vi "Create_Tree_PN.vi"(4 "Triangles":T3[](array[typedef]), 5 "Sf":dbl=0.6, 6 "dq":dbl=0.3927, 7 "L0":dbl=1.0, 8 "Pad":dbl=1.01) -> (0 "Mesh bounds":T1, 1 "Node stack size history":i32[](array[numeric]), 2 "All nodes processed and processed without error":bool, 3 "TreeNodes out":T2[](array[typedef]))   [LabVIEW 2011]
uses:
  Triangle2D.ctl
  TreeNode2D.ctl
  TreeNode2D Input Cluster.ctl
  <vilib>/Utility/file.llb/Write To Spreadsheet File (I64).vi
panel:
  out "Node tree representation":cluster{dbl[], dbl[]}(graph)
  out "Node stack size history":i32[](graph)
  in  "stop":bool
  in  "TreeNodes":T2[](array[typedef])
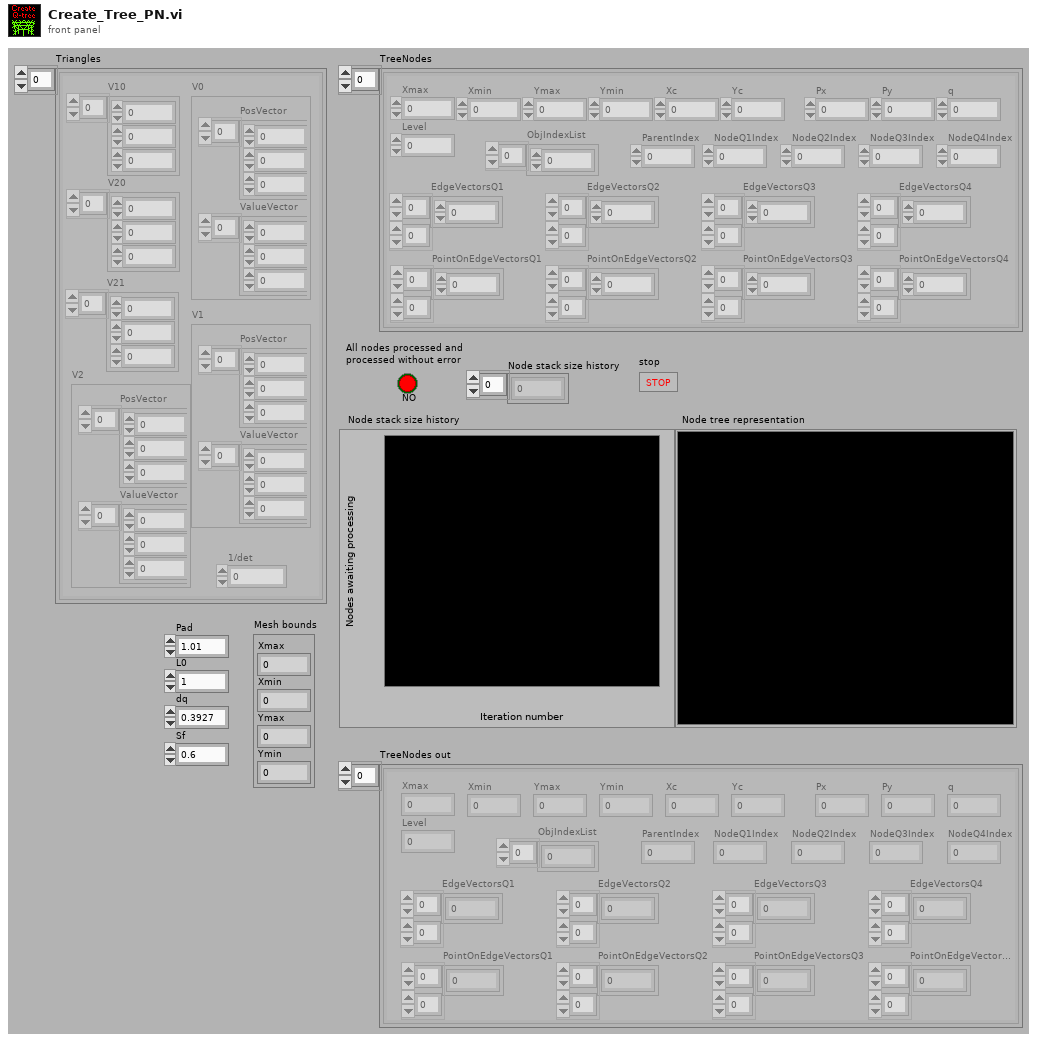
[diagram p1: front panel]
types:
  T1 = cluster{"Xmax":dbl, "Xmin":dbl, "Ymax":dbl, "Ymin":dbl}
  T2 = typedef "TreeNode2D.ctl" = cluster{"Xmax":dbl, "Xmin":dbl, "Ymax":dbl, "Ymin":dbl, "Xc":dbl, "Yc":dbl, "Px":dbl, "Py":dbl, "q":dbl, "Level":i32, "ObjIndexList":i32[], "ParentIndex":i32, "NodeQ1Index":i32, "NodeQ2Index":i32, "NodeQ3Index":i32, "NodeQ4Index":i32, "EdgeVectorsQ1":dbl[][], "EdgeVectorsQ2":dbl[][], "EdgeVectorsQ3":dbl[][], "EdgeVectorsQ4":dbl[][], "PointOnEdgeVectorsQ1":dbl[][], "PointOnEdgeVectorsQ2":dbl[][], "PointOnEdgeVectorsQ3":dbl[][], "PointOnEdgeVectorsQ4":dbl[][]}
  T3 = typedef "Triangle2D.ctl" = cluster{"V10":dbl[], "V20":dbl[], "1/det":dbl, "V0":cluster{"PosVector":dbl[], "ValueVector":dbl[]}, "V1":cluster{"PosVector":dbl[], "ValueVector":dbl[]}, "V2":cluster{"PosVector":dbl[], "ValueVector":dbl[]}, "V21":dbl[]}
  T4 = typedef "TreeNode2D Input Cluster.ctl" = cluster{"Xmax":dbl, "Xmin":dbl, "Ymax":dbl, "Ymin":dbl, "Xc":dbl, "Yc":dbl, "Px":dbl, "Py":dbl, "q":dbl, "Level":i32, "ObjIndexList":i32[], "ParentIndex":i32, "NodeQ1Index":i32, "NodeQ2Index":i32, "NodeQ3Index":i32, "NodeQ4Index":i32}
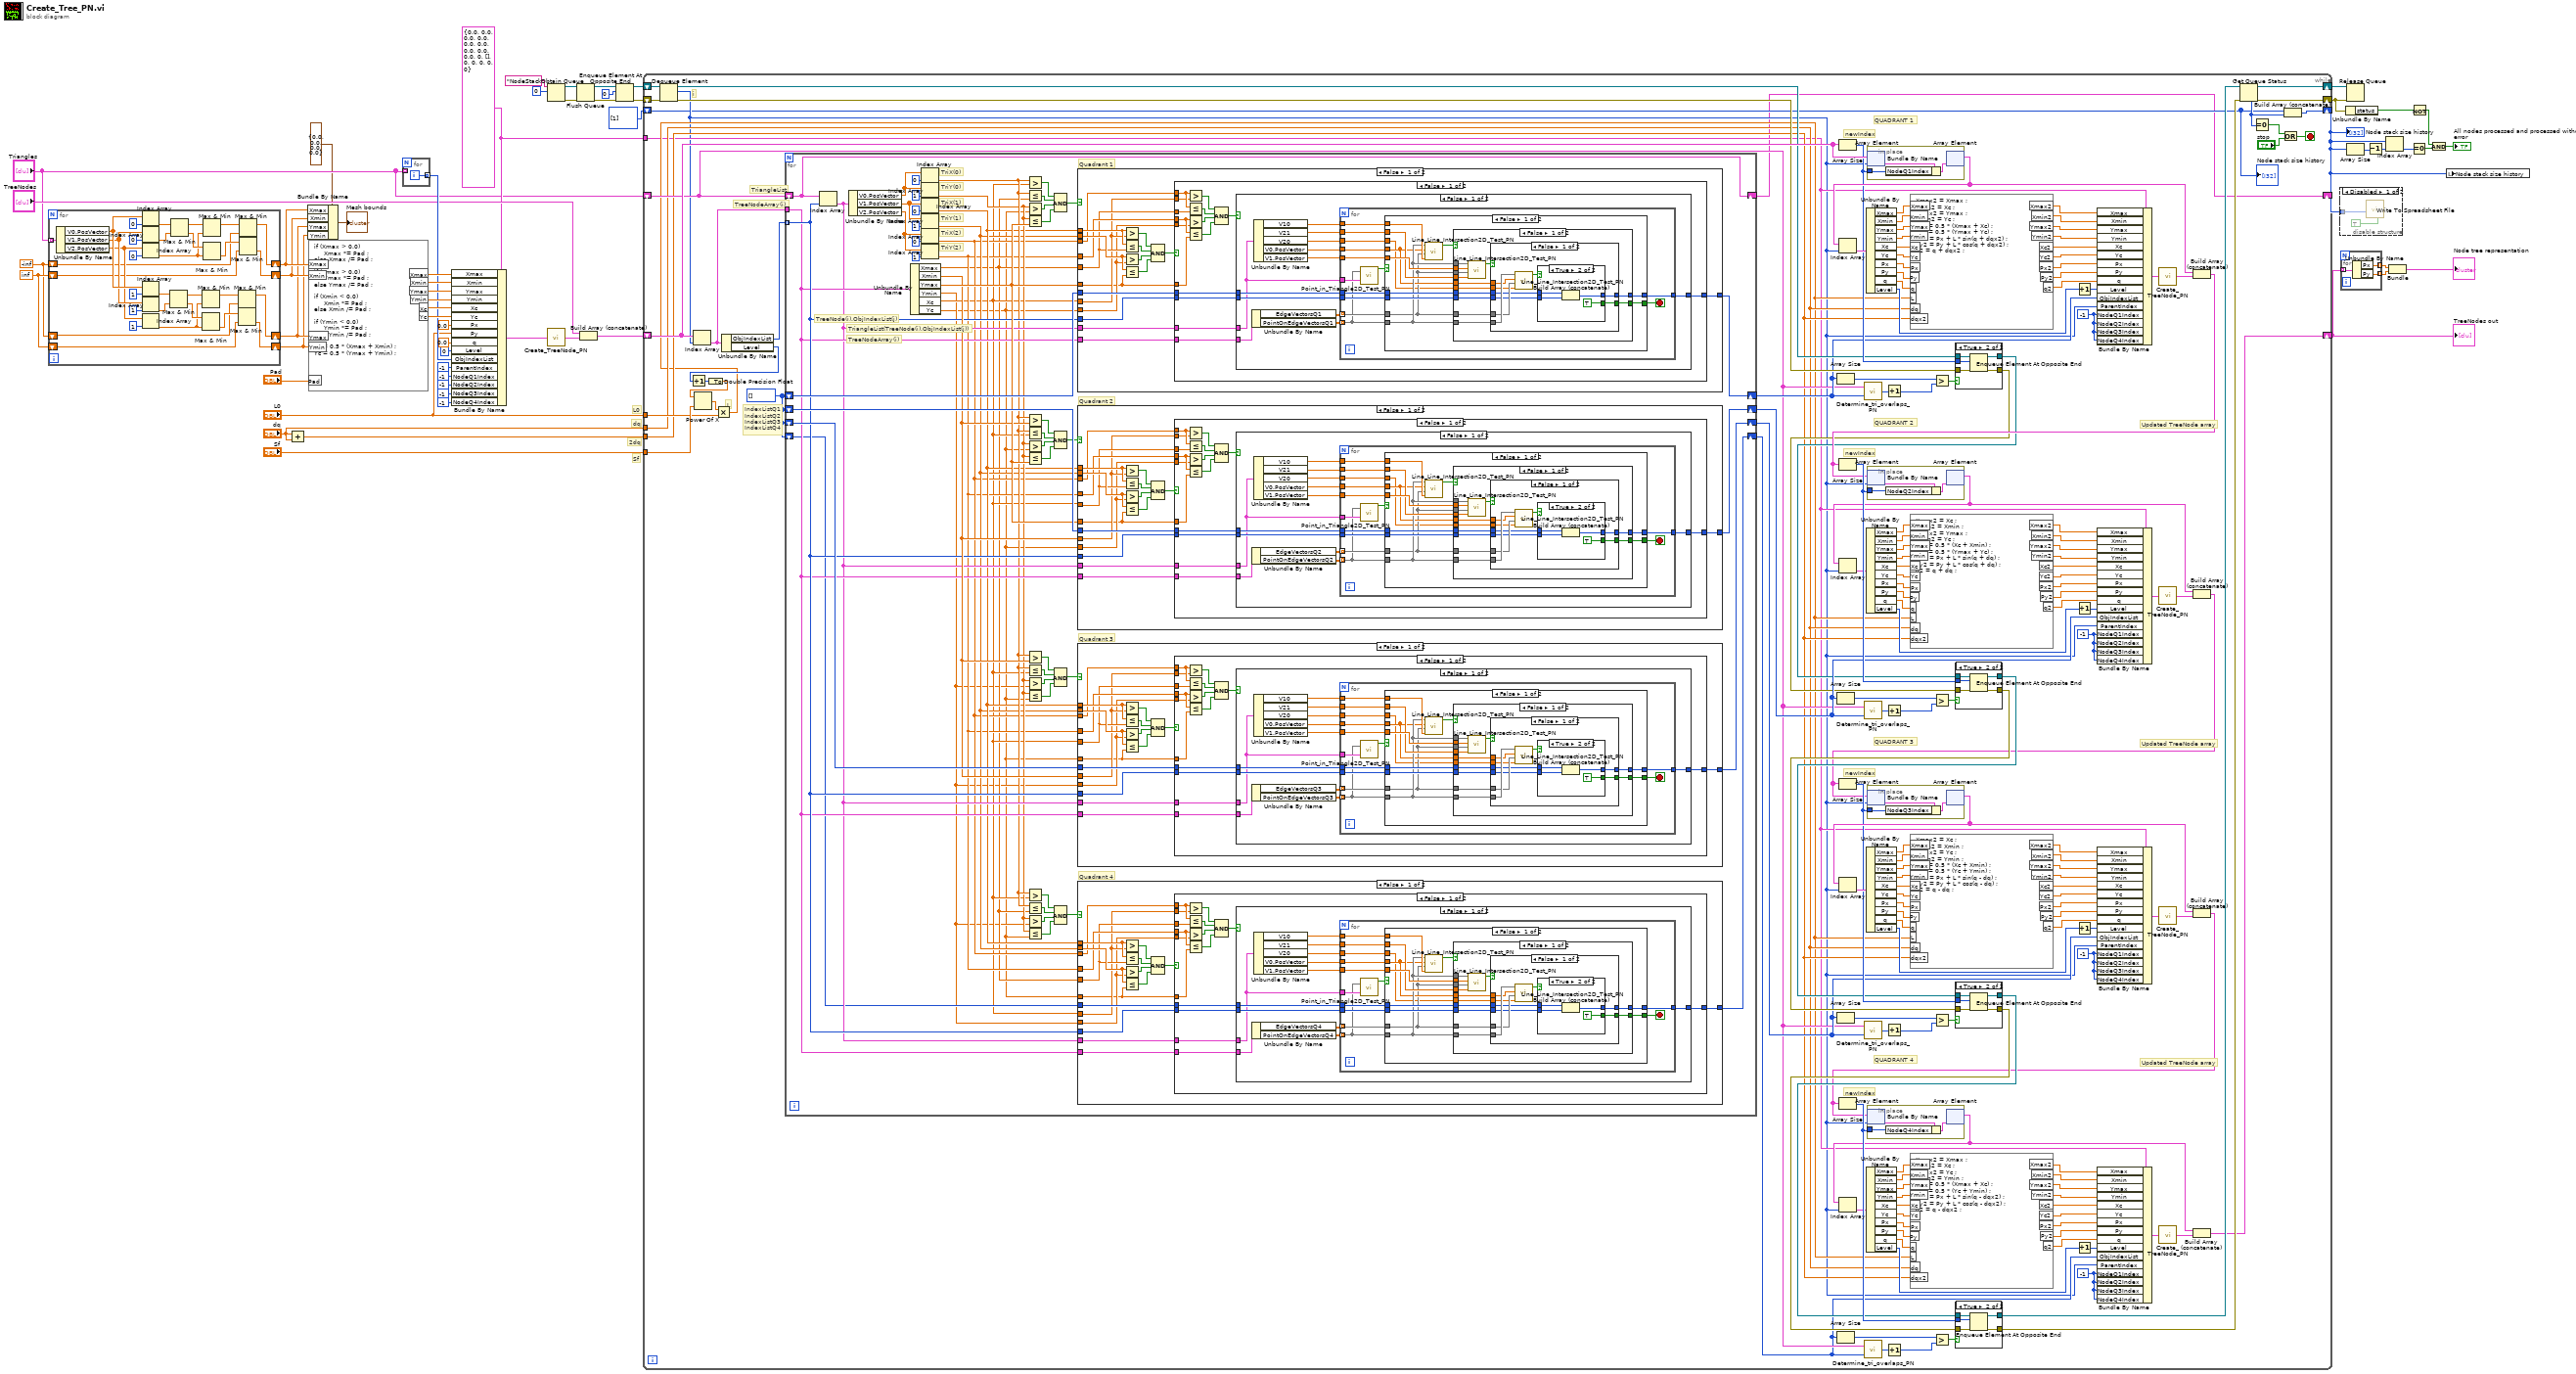
[diagram p0: block diagram]
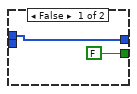
[diagram p7: hidden frame]
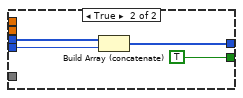
[diagram p8: hidden frame]
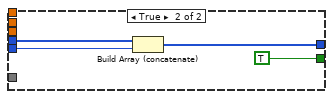
[diagram p9: hidden frame]
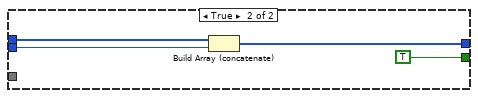
[diagram p10: hidden frame]
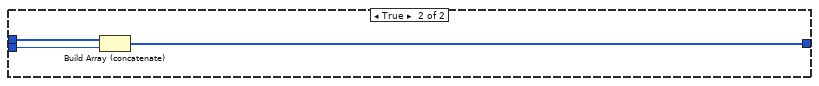
[diagram p11: hidden frame]
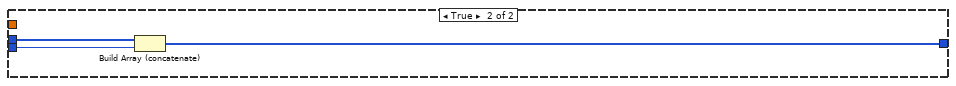
[diagram p12: hidden frame]
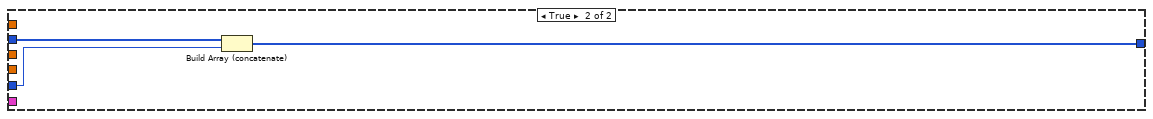
[diagram p13: hidden frame]
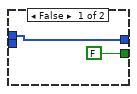
[diagram p14: hidden frame]
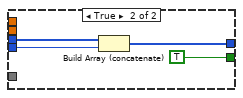
[diagram p15: hidden frame]
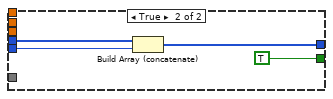
[diagram p16: hidden frame]
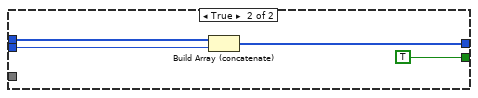
[diagram p17: hidden frame]
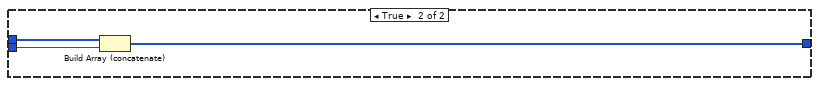
[diagram p18: hidden frame]
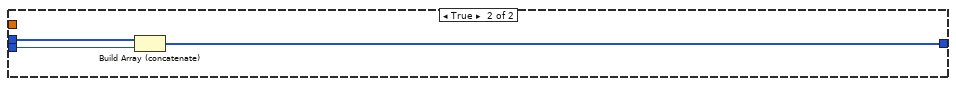
[diagram p19: hidden frame]
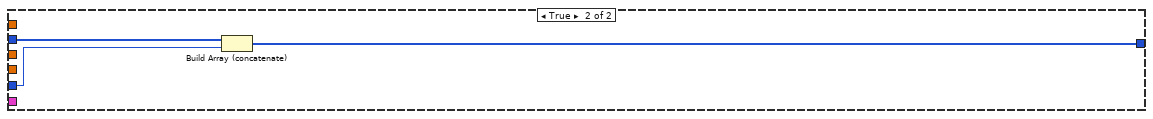
[diagram p20: hidden frame]
diagram:
  w8 = inf
  w7 = -inf
  w25 = T4 {"Xmax"=0.0, "Xmin"=0.0, "Ymax"=0.0, "Ymin"=0.0, "Xc"=0.0, "Yc"=0.0, "Px"=0.0, "Py"=0.0, "q"=0.0, "Level"=0, "ObjIndexList"=[], "ParentIndex"=0, "NodeQ1Index"=0, "NodeQ2Index"=0, "NodeQ3Index"=0, "NodeQ4Index"=0} ("Input cluster")
  # "Sf"
  # "L0"
  # "dq"
  # "2dq"
  n1 = for {
    tunnel: "Triangles" -> [w90] mode=indexing
    shift-right: [w72] -> w6
    shift-left: w7 -> [w73]
    shift-right: [w70] -> w5
    shift-left: w8 -> [w71]
    shift-right: [w60] -> w4
    shift-left: w7 -> [w62]
    shift-right: [w59] -> w3
    shift-left: w8 -> [w61]
    n2 = Unbundle By Name(w90) -> ("V0.PosVector"=w83:dbl[], "V1.PosVector"=w82:dbl[], "V2.PosVector"=w81:dbl[])
    n3 = Index Array(array=w83, index=0) -> (element=w80:dbl)
    n4 = Index Array(array=w82, index=0) -> (element=w79:dbl)
    n5 = Index Array(array=w81, index=0) -> (element=w76:dbl)
    n6 = Index Array(array=w83, index=1) -> (element=w65:dbl)
    n7 = Index Array(array=w82, index=1) -> (element=w64:dbl)
    n8 = Index Array(array=w81, index=1) -> (element=w63:dbl)
    n9 = Max & Min(x=w65, y=w64) -> (max(x,y)=w66:dbl, min(x,y)=w67:dbl)
    n10 = Max & Min(x=w80, y=w79) -> (max(x,y)=w78:dbl, min(x,y)=w77:dbl)
    n11 = Max & Min(x=w66, y=w63) -> (max(x,y)=w68:dbl)  [unwired: 1 out]
    n12 = Max & Min(x=w67, y=w63) -> (min(x,y)=w69:dbl)  [unwired: 1 out]
    n13 = Max & Min(x=w78, y=w76) -> (max(x,y)=w75:dbl)  [unwired: 1 out]
    n14 = Max & Min(x=w77, y=w76) -> (min(x,y)=w74:dbl)  [unwired: 1 out]
    n15 = Max & Min(x=w68, y=w62) -> (max(x,y)=w60:dbl)  [unwired: 1 out]
    n16 = Max & Min(x=w69, y=w61) -> (min(x,y)=w59:dbl)  [unwired: 1 out]
    n17 = Max & Min(x=w75, y=w73) -> (max(x,y)=w72:dbl)  [unwired: 1 out]
    n18 = Max & Min(x=w74, y=w71) -> (min(x,y)=w70:dbl)  [unwired: 1 out]
  }
  n19 = Add(x="dq", y="dq") -> (x+y=w27:dbl)
  n20 = Bundle By Name(cluster=T1 {"Xmax"=0.0, "Xmin"=0.0, "Ymax"=0.0, "Ymin"=0.0} ("Mesh bounds"), "Xmax"=w6, "Xmin"=w5, "Ymax"=w4, "Ymin"=w3) -> (→"Mesh bounds":T1)
  n21 = formula code="if (Xmax > 0.0)\n     Xmax *= Pad ;\nelse Xmax /= Pad ;\n\nif (Ymax > 0.0)\n     Ymax *= Pad ;\nelse Ymax /= Pad ;\n\nif (Xmin < 0.0)\n     Xmin *= Pad ;\nelse Xmin /= Pad ;\n\nif (Ymin < 0.0)\n     Ymin *= Pad ;\nelse Ymin /= Pad ;\n\nXc = 0.5 * (Xmax + Xmin) ;\nYc = 0.5 * (Ymax + Ymin) ;"("Xmax"=w6, "Xmin"=w5, "Ymax"=w4, "Ymin"=w3, "Pad"="Pad") -> ("Xmax"=w50:dbl, "Xmin"=w51:dbl, "Ymax"=w52:dbl, "Ymin"=w53:dbl, "Xc"=w55:dbl, "Yc"=w54:dbl)
  n22 = for {
    tunnel: "Triangles" -> [_] mode=indexing
    tunnel: [w91] -> w40 mode=indexing
    i -> [w91]
  }
  n23 = Bundle By Name(cluster=w25, "Xmax"=w50, "Xmin"=w51, "Ymax"=w52, "Ymin"=w53, "Xc"=w55, "Yc"=w54, "Px"=0.0, "Py"="L0", "q"=0.0, "Level"=0, "ObjIndexList"=w40, "ParentIndex"=-1, "NodeQ1Index"=-1, "NodeQ2Index"=-1, "NodeQ3Index"=-1, "NodeQ4Index"=-1) -> (w39:T4)
  n24 = Obtain Queue(name (unnamed)="NodeStack", element data type=0) -> (queue out=w37:refnum<queue>, error out=w38:errorcluster)  [unwired: 3 in, 1 out]
  n25 = call "Create_TreeNode_PN.vi"("Input cluster"=w39) -> ("TreeNode out"=w33:T2)
  n26 = Flush Queue(queue=w37, error in (no error)=w38) -> (queue out=w35:refnum<queue>, error out=w36:errorcluster)  [unwired: 1 out]
  n27 = Build Array (concatenate)("TreeNodes", w33) -> (w30:T2[])
  n28 = Enqueue Element At Opposite End(queue=w35, element=0, error in (no error)=w36) -> (queue out=w32:refnum<queue>, error out=w31:errorcluster)  [unwired: 2 out]
  n29 = while {
    shift-right: [w94] -> w11
    shift-left: w30 -> [w245]
    shift-right: [w253] -> w23
    shift-left: w31 -> [w256]
    shift-right: [w254] -> w29
    shift-left: w32 -> [w255]
    tunnel: "dq" -> [w107]
    tunnel: w27 -> [w108]
    tunnel: "L0" -> [w247]
    tunnel: "Sf" -> [w249]
    tunnel: w25 -> [w105]
    shift-right: [w99] -> w10
    shift-left: i32[] [1] -> [w93]
    shift-right: [w92] -> _
    shift-left: "Triangles" -> [w112]
    stop <- w97 stop-if-true
    w136 = -1 ("NodeQ1Index")
    w153 = -1 ("NodeQ1Index")
    w204 = -1 ("NodeQ1Index")
    w221 = -1 ("NodeQ1Index")
    w251 = i32[] []
    # "Updated TreeNode array"
    # "QUADRANT 4"
    # "newIndex"
    # "Updated TreeNode array"
    # "QUADRANT 3"
    # "newIndex"
    # "Updated TreeNode array"
    # "QUADRANT 2"
    # "newIndex"
    # "i"
    # "QUADRANT 1"
    # "newIndex"
    # "L"
    # "IndexListQ1\nIndexListQ2\nIndexListQ3\nIndexListQ4"
    # "TreeNodeArray(i)"
    # "TriangleList"
    n30 = Dequeue Element(queue=w255, error in (no error)=w256) -> (queue out=w216:refnum<queue>, element=w103:i32, error out=w215:errorcluster)  [unwired: 1 in, 1 out]
    n31 = Index Array(array=w245, index=w103) -> (element=w95:T2)
    n32 = Unbundle By Name(w95) -> ("ObjIndexList"=w252:i32[], "Level"=w250:i32)
    n33 = Increment(x=w250) -> (x+1=w246:i32)
    n34 = To Double Precision Float(number=w246) -> (double precision float=w213:dbl)
    n35 = Power Of X(1:w249, 2:w213) -> (0:w248:dbl)
    n36 = Multiply(x=w248, y=w247) -> (x*y=w106:dbl)
    n37 = for {
      tunnel: w95 -> [w316]
      tunnel: w252 -> [w317] mode=indexing
      shift-right: [w334] -> w211
      shift-left: w251 -> [w335]
      shift-right: [w332] -> w180
      shift-left: w251 -> [w333]
      shift-right: [w324] -> w143
      shift-left: w251 -> [w325]
      shift-right: [w298] -> w104
      shift-left: w251 -> [w314]
      shift-right: [w297] -> w92
      shift-left: w112 -> [w297]
      # "Quadrant 4"
      # "Quadrant 3"
      # "Quadrant 2"
      # "TreeNodeArray(i)"
      # "TriangleList(TreeNode(i).ObjIndexList(j))"
      # "TreeNode(i).ObjIndexList(j)"
      # "Quadrant 1"
      # "TriY(2)"
      # "TriX(2)"
      # "TriY(1)"
      # "TriX(1)"
      # "TriY(0)"
      # "TriX(0)"
      # "j"
      n38 = Index Array(array=w297, index=w317) -> (element=w315:T3)
      n39 = Unbundle By Name(w315) -> ("V0.PosVector"=w349:dbl[], "V1.PosVector"=w344:dbl[], "V2.PosVector"=w341:dbl[])
      n40 = Unbundle By Name(w316) -> ("Xmax"=w301:dbl, "Xmin"=w318:dbl, "Ymax"=w326:dbl, "Ymin"=w300:dbl, "Xc"=w302:dbl, "Yc"=w299:dbl)
      n41 = Index Array(array=w349, index=0) -> (element=w308:dbl)
      n42 = Index Array(array=w349, index=1) -> (element=w307:dbl)
      n43 = Index Array(array=w344, index=0) -> (element=w306:dbl)
      n44 = Index Array(array=w344, index=1) -> (element=w305:dbl)
      n45 = Index Array(array=w341, index=0) -> (element=w304:dbl)
      n46 = Index Array(array=w341, index=1) -> (element=w303:dbl)
      n47 = Greater?(x=w308, y=w302) -> (0:w340:bool)
      n48 = Less Or Equal?(x=w308, y=w301) -> (x <= y?=w339:bool)
      n49 = Greater?(x=w307, y=w299) -> (0:w338:bool)
      n50 = Less Or Equal?(x=w307, y=w326) -> (x <= y?=w337:bool)
      n51 = Greater?(x=w308, y=w318) -> (0:w328:bool)
      n52 = Less Or Equal?(x=w308, y=w302) -> (x <= y?=w329:bool)
      n53 = Greater?(x=w307, y=w299) -> (0:w330:bool)
      n54 = Less Or Equal?(x=w307, y=w326) -> (x <= y?=w331:bool)
      n55 = Greater?(x=w308, y=w318) -> (0:w323:bool)
      n56 = Less Or Equal?(x=w308, y=w302) -> (x <= y?=w322:bool)
      n57 = Greater?(x=w307, y=w300) -> (0:w321:bool)
      n58 = Less Or Equal?(x=w307, y=w299) -> (x <= y?=w320:bool)
      n59 = Greater?(x=w308, y=w302) -> (0:w310:bool)
      n60 = Less Or Equal?(x=w308, y=w301) -> (x <= y?=w311:bool)
      n61 = Greater?(x=w307, y=w300) -> (0:w312:bool)
      n62 = Less Or Equal?(x=w307, y=w299) -> (x <= y?=w313:bool)
      n63 = Compound Arithmetic op=AND(w340, w339, w338, w337) -> (w336:bool)
      n64 = Compound Arithmetic op=AND(w328, w329, w330, w331) -> (w327:bool)
      n65 = Compound Arithmetic op=AND(w323, w322, w321, w320) -> (w319:bool)
      n66 = Compound Arithmetic op=AND(w310, w311, w312, w313) -> (w309:bool)
      n67 = case shown="False" w336 {
        tunnel: w306 -> [w723 _]
        tunnel: w305 -> [w722 _]
        tunnel: w304 -> [w717 _]
        tunnel: w303 -> [w716 _]
        tunnel: w335 -> [w720 w829]
        tunnel: [w718 w828] -> w334
        tunnel: w317 -> [w719 w827]
        tunnel: w302 -> [w714 _]
        tunnel: w299 -> [w713 _]
        tunnel: w326 -> [w712 _]
        tunnel: w301 -> [w715 _]
        tunnel: w315 -> [w710 _]
        tunnel: w316 -> [w711 _]
        frame False {
          n68 = Greater?(x=w723, y=w714) -> (0:w724:bool)
          n69 = Less Or Equal?(x=w723, y=w715) -> (x <= y?=w725:bool)
          n70 = Greater?(x=w722, y=w713) -> (0:w726:bool)
          n71 = Less Or Equal?(x=w722, y=w712) -> (x <= y?=w727:bool)
          n72 = Compound Arithmetic op=AND(w724, w725, w726, w727) -> (w721:bool)
          n73 = case shown="False" w721 {
            tunnel: w720 -> [w731 w826]
            tunnel: w719 -> [w730 w825]
            tunnel: [w732 w824] -> w718
            tunnel: w717 -> [w739 _]
            tunnel: w716 -> [w738 _]
            tunnel: w715 -> [w737 _]
            tunnel: w714 -> [w736 _]
            tunnel: w713 -> [w735 _]
            tunnel: w712 -> [w734 _]
            tunnel: w711 -> [w729 _]
            tunnel: w710 -> [w728 _]
            frame False {
              n74 = Greater?(x=w739, y=w736) -> (0:w743:bool)
              n75 = Less Or Equal?(x=w739, y=w737) -> (x <= y?=w742:bool)
              n76 = Greater?(x=w738, y=w735) -> (0:w741:bool)
              n77 = Less Or Equal?(x=w738, y=w734) -> (x <= y?=w740:bool)
              n78 = Compound Arithmetic op=AND(w743, w742, w741, w740) -> (w733:bool)
              n79 = case shown="False" w733 {
                tunnel: [w745 w823] -> w732
                tunnel: w731 -> [w747 w822]
                tunnel: w730 -> [w746 w821]
                tunnel: w729 -> [w755 _]
                tunnel: w728 -> [w744 _]
                frame False {
                  n80 = Unbundle By Name(w755) -> ("EdgeVectorsQ1"=w754:dbl[][], "PointOnEdgeVectorsQ1"=w748:dbl[][])
                  n81 = Unbundle By Name(w744) -> ("V10"=w753:dbl[], "V21"=w752:dbl[], "V20"=w751:dbl[], "V0.PosVector"=w750:dbl[], "V1.PosVector"=w749:dbl[])
                  n82 = for {
                    tunnel: w754 -> [w762] mode=indexing
                    tunnel: w753 -> [w756]
                    tunnel: w752 -> [w757]
                    tunnel: w751 -> [w758]
                    tunnel: w750 -> [w759]
                    tunnel: w749 -> [w760]
                    tunnel: w748 -> [w761] mode=indexing
                    tunnel: w747 -> [w768]
                    tunnel: w746 -> [w767]
                    tunnel: [w766] -> w745
                    tunnel: w744 -> [w764]
                    stop <- w765 stop-if-true
                    n83 = call "Point_in_Triangle2D_Test_PN.vi"("2D Point to Test"=w761, "Triangle2D"=w764) -> ("Point is in triangle"=w763:bool)  [unwired: 3 out]
                    n84 = case shown="False" w763 {
                      tunnel: w768 -> [w776 w820]
                      tunnel: w767 -> [w775 w819]
                      tunnel: [w777 w818] -> w766
                      tunnel: [w778 TRUE] -> w765
                      tunnel: w762 -> [w770 _]
                      tunnel: w761 -> [w772 _]
                      tunnel: w760 -> [w774 _]
                      tunnel: w759 -> [w771 _]
                      tunnel: w758 -> [w769 _]
                      tunnel: w757 -> [w773 _]
                      tunnel: w756 -> [w780 _]
                      frame False {
                        n85 = call "Line_Line_Intersection2D_Test_PN.vi"("2D Dir. Vect. of Line 2 (not unit)"=w780, "2D Dir. Vect. of Line 1 (not unit)"=w770, "2D Point on Line 2"=w771, "2D Point on Line 1"=w772) -> ("Lines Intersect"=w779:bool)  [unwired: 2 out]
                        n86 = case shown="False" w779 {
                          tunnel: [w788 TRUE] -> w778
                          tunnel: [w785 w815] -> w777
                          tunnel: w776 -> [w787 w814]
                          tunnel: w775 -> [w786 w813]
                          tunnel: w772 -> [w793 _]
                          tunnel: w774 -> [w792 _]
                          tunnel: w770 -> [w791 _]
                          tunnel: w773 -> [w790 _]
                          tunnel: w772 -> [w784 _]
                          tunnel: w771 -> [w783 _]
                          tunnel: w770 -> [w782 _]
                          tunnel: w769 -> [w781 _]
                          frame False {
                            n87 = call "Line_Line_Intersection2D_Test_PN.vi"("2D Dir. Vect. of Line 2 (not unit)"=w790, "2D Dir. Vect. of Line 1 (not unit)"=w791, "2D Point on Line 2"=w792, "2D Point on Line 1"=w793) -> ("Lines Intersect"=w789:bool)  [unwired: 2 out]
                            n88 = case shown="False" w789 {
                              tunnel: [w797 TRUE] -> w788
                              tunnel: w787 -> [w796 w811]
                              tunnel: w786 -> [w795 w810]
                              tunnel: [w794 w809] -> w785
                              tunnel: w784 -> [w802 _]
                              tunnel: w783 -> [w801 _]
                              tunnel: w782 -> [w800 _]
                              tunnel: w781 -> [w799 _]
                              frame False {
                                n89 = call "Line_Line_Intersection2D_Test_PN.vi"("2D Dir. Vect. of Line 2 (not unit)"=w799, "2D Dir. Vect. of Line 1 (not unit)"=w800, "2D Point on Line 2"=w801, "2D Point on Line 1"=w802) -> ("Lines Intersect"=w798:bool)  [unwired: 2 out]
                                n90 = case shown="True" w798 {
                                tunnel: [FALSE TRUE] -> w797
                                tunnel: w796 -> [w804 w807]
                                tunnel: w795 -> [_ w806]
                                tunnel: [w804 w805] -> w794
                                frame False {
                                }
                                frame True {
                                n91 = Build Array (concatenate)(w807, w806) -> (w805:i32[])
                                }
                                }
                              }
                              frame True {
                                n92 = Build Array (concatenate)(w811, w810) -> (w809:i32[])
                              }
                            }
                          }
                          frame True {
                            n93 = Build Array (concatenate)(w814, w813) -> (w815:i32[])
                          }
                        }
                      }
                      frame True {
                        n94 = Build Array (concatenate)(w820, w819) -> (w818:i32[])
                      }
                    }
                  }
                }
                frame True {
                  n95 = Build Array (concatenate)(w822, w821) -> (w823:i32[])
                }
              }
            }
            frame True {
              n96 = Build Array (concatenate)(w826, w825) -> (w824:i32[])
            }
          }
        }
        frame True {
          n97 = Build Array (concatenate)(w829, w827) -> (w828:i32[])
        }
      }
      n98 = case shown="False" w327 {
        tunnel: w306 -> [w603 _]
        tunnel: w305 -> [w602 _]
        tunnel: w304 -> [w597 _]
        tunnel: w303 -> [w596 _]
        tunnel: w333 -> [w600 w709]
        tunnel: [w598 w708] -> w332
        tunnel: w317 -> [w599 w707]
        tunnel: w318 -> [w594 _]
        tunnel: w299 -> [w593 _]
        tunnel: w326 -> [w592 _]
        tunnel: w302 -> [w595 _]
        tunnel: w315 -> [w590 _]
        tunnel: w316 -> [w591 _]
        frame False {
          n99 = Greater?(x=w603, y=w594) -> (0:w604:bool)
          n100 = Less Or Equal?(x=w603, y=w595) -> (x <= y?=w605:bool)
          n101 = Greater?(x=w602, y=w593) -> (0:w606:bool)
          n102 = Less Or Equal?(x=w602, y=w592) -> (x <= y?=w607:bool)
          n103 = Compound Arithmetic op=AND(w604, w605, w606, w607) -> (w601:bool)
          n104 = case shown="False" w601 {
            tunnel: w600 -> [w611 w706]
            tunnel: w599 -> [w610 w705]
            tunnel: [w612 w704] -> w598
            tunnel: w597 -> [w619 _]
            tunnel: w596 -> [w618 _]
            tunnel: w595 -> [w617 _]
            tunnel: w594 -> [w616 _]
            tunnel: w593 -> [w615 _]
            tunnel: w592 -> [w614 _]
            tunnel: w591 -> [w609 _]
            tunnel: w590 -> [w608 _]
            frame False {
              n105 = Greater?(x=w619, y=w616) -> (0:w623:bool)
              n106 = Less Or Equal?(x=w619, y=w617) -> (x <= y?=w622:bool)
              n107 = Greater?(x=w618, y=w615) -> (0:w621:bool)
              n108 = Less Or Equal?(x=w618, y=w614) -> (x <= y?=w620:bool)
              n109 = Compound Arithmetic op=AND(w623, w622, w621, w620) -> (w613:bool)
              n110 = case shown="False" w613 {
                tunnel: [w625 w703] -> w612
                tunnel: w611 -> [w627 w702]
                tunnel: w610 -> [w626 w701]
                tunnel: w609 -> [w635 _]
                tunnel: w608 -> [w624 _]
                frame False {
                  n111 = Unbundle By Name(w635) -> ("EdgeVectorsQ2"=w634:dbl[][], "PointOnEdgeVectorsQ2"=w628:dbl[][])
                  n112 = Unbundle By Name(w624) -> ("V10"=w633:dbl[], "V21"=w632:dbl[], "V20"=w631:dbl[], "V0.PosVector"=w630:dbl[], "V1.PosVector"=w629:dbl[])
                  n113 = for {
                    tunnel: w634 -> [w642] mode=indexing
                    tunnel: w633 -> [w636]
                    tunnel: w632 -> [w637]
                    tunnel: w631 -> [w638]
                    tunnel: w630 -> [w639]
                    tunnel: w629 -> [w640]
                    tunnel: w628 -> [w641] mode=indexing
                    tunnel: w627 -> [w648]
                    tunnel: w626 -> [w647]
                    tunnel: [w646] -> w625
                    tunnel: w624 -> [w644]
                    stop <- w645 stop-if-true
                    n114 = call "Point_in_Triangle2D_Test_PN.vi"("2D Point to Test"=w641, "Triangle2D"=w644) -> ("Point is in triangle"=w643:bool)  [unwired: 3 out]
                    n115 = case shown="False" w643 {
                      tunnel: w648 -> [w656 w700]
                      tunnel: w647 -> [w655 w699]
                      tunnel: [w657 w698] -> w646
                      tunnel: [w658 TRUE] -> w645
                      tunnel: w642 -> [w650 _]
                      tunnel: w641 -> [w652 _]
                      tunnel: w640 -> [w654 _]
                      tunnel: w639 -> [w651 _]
                      tunnel: w638 -> [w649 _]
                      tunnel: w637 -> [w653 _]
                      tunnel: w636 -> [w660 _]
                      frame False {
                        n116 = call "Line_Line_Intersection2D_Test_PN.vi"("2D Dir. Vect. of Line 2 (not unit)"=w660, "2D Dir. Vect. of Line 1 (not unit)"=w650, "2D Point on Line 2"=w651, "2D Point on Line 1"=w652) -> ("Lines Intersect"=w659:bool)  [unwired: 2 out]
                        n117 = case shown="False" w659 {
                          tunnel: [w668 TRUE] -> w658
                          tunnel: [w665 w695] -> w657
                          tunnel: w656 -> [w667 w694]
                          tunnel: w655 -> [w666 w693]
                          tunnel: w652 -> [w673 _]
                          tunnel: w654 -> [w672 _]
                          tunnel: w650 -> [w671 _]
                          tunnel: w653 -> [w670 _]
                          tunnel: w652 -> [w664 _]
                          tunnel: w651 -> [w663 _]
                          tunnel: w650 -> [w662 _]
                          tunnel: w649 -> [w661 _]
                          frame False {
                            n118 = call "Line_Line_Intersection2D_Test_PN.vi"("2D Dir. Vect. of Line 2 (not unit)"=w670, "2D Dir. Vect. of Line 1 (not unit)"=w671, "2D Point on Line 2"=w672, "2D Point on Line 1"=w673) -> ("Lines Intersect"=w669:bool)  [unwired: 2 out]
                            n119 = case shown="False" w669 {
                              tunnel: [w677 TRUE] -> w668
                              tunnel: w667 -> [w676 w691]
                              tunnel: w666 -> [w675 w690]
                              tunnel: [w674 w689] -> w665
                              tunnel: w664 -> [w682 _]
                              tunnel: w663 -> [w681 _]
                              tunnel: w662 -> [w680 _]
                              tunnel: w661 -> [w679 _]
                              frame False {
                                n120 = call "Line_Line_Intersection2D_Test_PN.vi"("2D Dir. Vect. of Line 2 (not unit)"=w679, "2D Dir. Vect. of Line 1 (not unit)"=w680, "2D Point on Line 2"=w681, "2D Point on Line 1"=w682) -> ("Lines Intersect"=w678:bool)  [unwired: 2 out]
                                n121 = case shown="True" w678 {
                                tunnel: [FALSE TRUE] -> w677
                                tunnel: w676 -> [w684 w687]
                                tunnel: w675 -> [_ w686]
                                tunnel: [w684 w685] -> w674
                                frame False {
                                }
                                frame True {
                                n122 = Build Array (concatenate)(w687, w686) -> (w685:i32[])
                                }
                                }
                              }
                              frame True {
                                n123 = Build Array (concatenate)(w691, w690) -> (w689:i32[])
                              }
                            }
                          }
                          frame True {
                            n124 = Build Array (concatenate)(w694, w693) -> (w695:i32[])
                          }
                        }
                      }
                      frame True {
                        n125 = Build Array (concatenate)(w700, w699) -> (w698:i32[])
                      }
                    }
                  }
                }
                frame True {
                  n126 = Build Array (concatenate)(w702, w701) -> (w703:i32[])
                }
              }
            }
            frame True {
              n127 = Build Array (concatenate)(w706, w705) -> (w704:i32[])
            }
          }
        }
        frame True {
          n128 = Build Array (concatenate)(w709, w707) -> (w708:i32[])
        }
      }
      n129 = case shown="False" w319 {
        tunnel: w306 -> [w483 _]
        tunnel: w305 -> [w482 _]
        tunnel: w304 -> [w477 _]
        tunnel: w303 -> [w476 _]
        tunnel: w325 -> [w480 w589]
        tunnel: [w478 w588] -> w324
        tunnel: w317 -> [w479 w587]
        tunnel: w318 -> [w474 _]
        tunnel: w300 -> [w473 _]
        tunnel: w299 -> [w472 _]
        tunnel: w302 -> [w475 _]
        tunnel: w315 -> [w470 _]
        tunnel: w316 -> [w471 _]
        frame False {
          n130 = Greater?(x=w483, y=w474) -> (0:w484:bool)
          n131 = Less Or Equal?(x=w483, y=w475) -> (x <= y?=w485:bool)
          n132 = Greater?(x=w482, y=w473) -> (0:w486:bool)
          n133 = Less Or Equal?(x=w482, y=w472) -> (x <= y?=w487:bool)
          n134 = Compound Arithmetic op=AND(w484, w485, w486, w487) -> (w481:bool)
          n135 = case shown="False" w481 {
            tunnel: w480 -> [w491 w586]
            tunnel: w479 -> [w490 w585]
            tunnel: [w492 w584] -> w478
            tunnel: w477 -> [w499 _]
            tunnel: w476 -> [w498 _]
            tunnel: w475 -> [w497 _]
            tunnel: w474 -> [w496 _]
            tunnel: w473 -> [w495 _]
            tunnel: w472 -> [w494 _]
            tunnel: w471 -> [w489 _]
            tunnel: w470 -> [w488 _]
            frame False {
              n136 = Greater?(x=w499, y=w496) -> (0:w503:bool)
              n137 = Less Or Equal?(x=w499, y=w497) -> (x <= y?=w502:bool)
              n138 = Greater?(x=w498, y=w495) -> (0:w501:bool)
              n139 = Less Or Equal?(x=w498, y=w494) -> (x <= y?=w500:bool)
              n140 = Compound Arithmetic op=AND(w503, w502, w501, w500) -> (w493:bool)
              n141 = case shown="False" w493 {
                tunnel: [w505 w583] -> w492
                tunnel: w491 -> [w507 w582]
                tunnel: w490 -> [w506 w581]
                tunnel: w489 -> [w515 _]
                tunnel: w488 -> [w504 _]
                frame False {
                  n142 = Unbundle By Name(w515) -> ("EdgeVectorsQ3"=w514:dbl[][], "PointOnEdgeVectorsQ3"=w508:dbl[][])
                  n143 = Unbundle By Name(w504) -> ("V10"=w513:dbl[], "V21"=w512:dbl[], "V20"=w511:dbl[], "V0.PosVector"=w510:dbl[], "V1.PosVector"=w509:dbl[])
                  n144 = for {
                    tunnel: w514 -> [w522] mode=indexing
                    tunnel: w513 -> [w516]
                    tunnel: w512 -> [w517]
                    tunnel: w511 -> [w518]
                    tunnel: w510 -> [w519]
                    tunnel: w509 -> [w520]
                    tunnel: w508 -> [w521] mode=indexing
                    tunnel: w507 -> [w528]
                    tunnel: w506 -> [w527]
                    tunnel: [w526] -> w505
                    tunnel: w504 -> [w524]
                    stop <- w525 stop-if-true
                    n145 = call "Point_in_Triangle2D_Test_PN.vi"("2D Point to Test"=w521, "Triangle2D"=w524) -> ("Point is in triangle"=w523:bool)  [unwired: 3 out]
                    n146 = case shown="False" w523 {
                      tunnel: w528 -> [w536 w580]
                      tunnel: w527 -> [w535 w579]
                      tunnel: [w537 w578] -> w526
                      tunnel: [w538 TRUE] -> w525
                      tunnel: w522 -> [w530 _]
                      tunnel: w521 -> [w532 _]
                      tunnel: w520 -> [w534 _]
                      tunnel: w519 -> [w531 _]
                      tunnel: w518 -> [w529 _]
                      tunnel: w517 -> [w533 _]
                      tunnel: w516 -> [w540 _]
                      frame False {
                        n147 = call "Line_Line_Intersection2D_Test_PN.vi"("2D Dir. Vect. of Line 2 (not unit)"=w540, "2D Dir. Vect. of Line 1 (not unit)"=w530, "2D Point on Line 2"=w531, "2D Point on Line 1"=w532) -> ("Lines Intersect"=w539:bool)  [unwired: 2 out]
                        n148 = case shown="False" w539 {
                          tunnel: [w548 TRUE] -> w538
                          tunnel: [w545 w575] -> w537
                          tunnel: w536 -> [w547 w574]
                          tunnel: w535 -> [w546 w573]
                          tunnel: w532 -> [w553 _]
                          tunnel: w534 -> [w552 _]
                          tunnel: w530 -> [w551 _]
                          tunnel: w533 -> [w550 _]
                          tunnel: w532 -> [w544 _]
                          tunnel: w531 -> [w543 _]
                          tunnel: w530 -> [w542 _]
                          tunnel: w529 -> [w541 _]
                          frame False {
                            n149 = call "Line_Line_Intersection2D_Test_PN.vi"("2D Dir. Vect. of Line 2 (not unit)"=w550, "2D Dir. Vect. of Line 1 (not unit)"=w551, "2D Point on Line 2"=w552, "2D Point on Line 1"=w553) -> ("Lines Intersect"=w549:bool)  [unwired: 2 out]
                            n150 = case shown="False" w549 {
                              tunnel: [w557 TRUE] -> w548
                              tunnel: w547 -> [w556 w571]
                              tunnel: w546 -> [w555 w570]
                              tunnel: [w554 w569] -> w545
                              tunnel: w544 -> [w562 _]
                              tunnel: w543 -> [w561 _]
                              tunnel: w542 -> [w560 _]
                              tunnel: w541 -> [w559 _]
                              frame False {
                                n151 = call "Line_Line_Intersection2D_Test_PN.vi"("2D Dir. Vect. of Line 2 (not unit)"=w559, "2D Dir. Vect. of Line 1 (not unit)"=w560, "2D Point on Line 2"=w561, "2D Point on Line 1"=w562) -> ("Lines Intersect"=w558:bool)  [unwired: 2 out]
                                n152 = case shown="True" w558 {
                                tunnel: [FALSE TRUE] -> w557
                                tunnel: w556 -> [w564 w567]
                                tunnel: w555 -> [_ w566]
                                tunnel: [w564 w565] -> w554
                                frame False {
                                }
                                frame True {
                                n153 = Build Array (concatenate)(w567, w566) -> (w565:i32[])
                                }
                                }
                              }
                              frame True {
                                n154 = Build Array (concatenate)(w571, w570) -> (w569:i32[])
                              }
                            }
                          }
                          frame True {
                            n155 = Build Array (concatenate)(w574, w573) -> (w575:i32[])
                          }
                        }
                      }
                      frame True {
                        n156 = Build Array (concatenate)(w580, w579) -> (w578:i32[])
                      }
                    }
                  }
                }
                frame True {
                  n157 = Build Array (concatenate)(w582, w581) -> (w583:i32[])
                }
              }
            }
            frame True {
              n158 = Build Array (concatenate)(w586, w585) -> (w584:i32[])
            }
          }
        }
        frame True {
          n159 = Build Array (concatenate)(w589, w587) -> (w588:i32[])
        }
      }
      n160 = case shown="False" w309 {
        tunnel: w306 -> [w363 _]
        tunnel: w305 -> [w362 _]
        tunnel: w304 -> [w357 _]
        tunnel: w303 -> [w356 _]
        tunnel: w314 -> [w360 w469]
        tunnel: [w358 w468] -> w298
        tunnel: w317 -> [w359 w467]
        tunnel: w302 -> [w354 _]
        tunnel: w300 -> [w353 _]
        tunnel: w299 -> [w352 _]
        tunnel: w301 -> [w355 _]
        tunnel: w315 -> [w350 _]
        tunnel: w316 -> [w351 _]
        frame False {
          n161 = Greater?(x=w363, y=w354) -> (0:w364:bool)
          n162 = Less Or Equal?(x=w363, y=w355) -> (x <= y?=w365:bool)
          n163 = Greater?(x=w362, y=w353) -> (0:w366:bool)
          n164 = Less Or Equal?(x=w362, y=w352) -> (x <= y?=w367:bool)
          n165 = Compound Arithmetic op=AND(w364, w365, w366, w367) -> (w361:bool)
          n166 = case shown="False" w361 {
            tunnel: w360 -> [w371 w466]
            tunnel: w359 -> [w370 w465]
            tunnel: [w372 w464] -> w358
            tunnel: w357 -> [w379 _]
            tunnel: w356 -> [w378 _]
            tunnel: w355 -> [w377 _]
            tunnel: w354 -> [w376 _]
            tunnel: w353 -> [w375 _]
            tunnel: w352 -> [w374 _]
            tunnel: w351 -> [w369 _]
            tunnel: w350 -> [w368 _]
            frame False {
              n167 = Greater?(x=w379, y=w376) -> (0:w383:bool)
              n168 = Less Or Equal?(x=w379, y=w377) -> (x <= y?=w382:bool)
              n169 = Greater?(x=w378, y=w375) -> (0:w381:bool)
              n170 = Less Or Equal?(x=w378, y=w374) -> (x <= y?=w380:bool)
              n171 = Compound Arithmetic op=AND(w383, w382, w381, w380) -> (w373:bool)
              n172 = case shown="False" w373 {
                tunnel: [w385 w463] -> w372
                tunnel: w371 -> [w387 w462]
                tunnel: w370 -> [w386 w461]
                tunnel: w369 -> [w395 _]
                tunnel: w368 -> [w384 _]
                frame False {
                  n173 = Unbundle By Name(w395) -> ("EdgeVectorsQ4"=w394:dbl[][], "PointOnEdgeVectorsQ4"=w388:dbl[][])
                  n174 = Unbundle By Name(w384) -> ("V10"=w393:dbl[], "V21"=w392:dbl[], "V20"=w391:dbl[], "V0.PosVector"=w390:dbl[], "V1.PosVector"=w389:dbl[])
                  n175 = for {
                    tunnel: w394 -> [w402] mode=indexing
                    tunnel: w393 -> [w396]
                    tunnel: w392 -> [w397]
                    tunnel: w391 -> [w398]
                    tunnel: w390 -> [w399]
                    tunnel: w389 -> [w400]
                    tunnel: w388 -> [w401] mode=indexing
                    tunnel: w387 -> [w408]
                    tunnel: w386 -> [w407]
                    tunnel: [w406] -> w385
                    tunnel: w384 -> [w404]
                    stop <- w405 stop-if-true
                    n176 = call "Point_in_Triangle2D_Test_PN.vi"("2D Point to Test"=w401, "Triangle2D"=w404) -> ("Point is in triangle"=w403:bool)  [unwired: 3 out]
                    n177 = case shown="False" w403 {
                      tunnel: w408 -> [w416 w460]
                      tunnel: w407 -> [w415 w459]
                      tunnel: [w417 w458] -> w406
                      tunnel: [w418 TRUE] -> w405
                      tunnel: w402 -> [w410 _]
                      tunnel: w401 -> [w412 _]
                      tunnel: w400 -> [w414 _]
                      tunnel: w399 -> [w411 _]
                      tunnel: w398 -> [w409 _]
                      tunnel: w397 -> [w413 _]
                      tunnel: w396 -> [w420 _]
                      frame False {
                        n178 = call "Line_Line_Intersection2D_Test_PN.vi"("2D Dir. Vect. of Line 2 (not unit)"=w420, "2D Dir. Vect. of Line 1 (not unit)"=w410, "2D Point on Line 2"=w411, "2D Point on Line 1"=w412) -> ("Lines Intersect"=w419:bool)  [unwired: 2 out]
                        n179 = case shown="False" w419 {
                          tunnel: [w428 TRUE] -> w418
                          tunnel: [w425 w455] -> w417
                          tunnel: w416 -> [w427 w454]
                          tunnel: w415 -> [w426 w453]
                          tunnel: w412 -> [w433 _]
                          tunnel: w414 -> [w432 _]
                          tunnel: w410 -> [w431 _]
                          tunnel: w413 -> [w430 _]
                          tunnel: w412 -> [w424 _]
                          tunnel: w411 -> [w423 _]
                          tunnel: w410 -> [w422 _]
                          tunnel: w409 -> [w421 _]
                          frame False {
                            n180 = call "Line_Line_Intersection2D_Test_PN.vi"("2D Dir. Vect. of Line 2 (not unit)"=w430, "2D Dir. Vect. of Line 1 (not unit)"=w431, "2D Point on Line 2"=w432, "2D Point on Line 1"=w433) -> ("Lines Intersect"=w429:bool)  [unwired: 2 out]
                            n181 = case shown="False" w429 {
                              tunnel: [w437 TRUE] -> w428
                              tunnel: w427 -> [w436 w451]
                              tunnel: w426 -> [w435 w450]
                              tunnel: [w434 w449] -> w425
                              tunnel: w424 -> [w442 _]
                              tunnel: w423 -> [w441 _]
                              tunnel: w422 -> [w440 _]
                              tunnel: w421 -> [w439 _]
                              frame False {
                                n182 = call "Line_Line_Intersection2D_Test_PN.vi"("2D Dir. Vect. of Line 2 (not unit)"=w439, "2D Dir. Vect. of Line 1 (not unit)"=w440, "2D Point on Line 2"=w441, "2D Point on Line 1"=w442) -> ("Lines Intersect"=w438:bool)  [unwired: 2 out]
                                n183 = case shown="True" w438 {
                                tunnel: [FALSE TRUE] -> w437
                                tunnel: w436 -> [w444 w447]
                                tunnel: w435 -> [_ w446]
                                tunnel: [w444 w445] -> w434
                                frame False {
                                }
                                frame True {
                                n184 = Build Array (concatenate)(w447, w446) -> (w445:i32[])
                                }
                                }
                              }
                              frame True {
                                n185 = Build Array (concatenate)(w451, w450) -> (w449:i32[])
                              }
                            }
                          }
                          frame True {
                            n186 = Build Array (concatenate)(w454, w453) -> (w455:i32[])
                          }
                        }
                      }
                      frame True {
                        n187 = Build Array (concatenate)(w460, w459) -> (w458:i32[])
                      }
                    }
                  }
                }
                frame True {
                  n188 = Build Array (concatenate)(w462, w461) -> (w463:i32[])
                }
              }
            }
            frame True {
              n189 = Build Array (concatenate)(w466, w465) -> (w464:i32[])
            }
          }
        }
        frame True {
          n190 = Build Array (concatenate)(w469, w467) -> (w468:i32[])
        }
      }
    }
    n191 = Array Size(array=w211) -> (size(s)=w220:i32)
    n192 = Array Size(array=w180) -> (size(s)=w205:i32)
    n193 = Array Size(array=w143) -> (size(s)=w152:i32)
    n194 = Array Size(array=w104) -> (size(s)=w137:i32)
    n195 = Array Size(array=w245) -> (size(s)=w217:i32)
    n196 = call "Determine_tri_overlaps_PN.vi"("Indices to check"=w211, "All triangles"=w112) -> ("Max. no. of intersections"=w212:i32)
    n197 = call "Determine_tri_overlaps_PN.vi"("Indices to check"=w180, "All triangles"=w112) -> ("Max. no. of intersections"=w210:i32)
    n198 = call "Determine_tri_overlaps_PN.vi"("Indices to check"=w143, "All triangles"=w112) -> ("Max. no. of intersections"=w147:i32)
    n199 = call "Determine_tri_overlaps_PN.vi"("Indices to check"=w104, "All triangles"=w112) -> ("Max. no. of intersections"=w142:i32)
    n200 = in-place {
      in-place-border: w217 -> [w295]
      n201 = in-place-array #1(w245, w103) -> (w296:T2)
      n202 = Bundle By Name(cluster=w296, "NodeQ1Index"=w295) -> (w294:T2)
      n203 = in-place-array #1(w294) -> (w241:T2[])  [unwired: 1 out]
    }
    n204 = Index Array(array=w241, index=w103) -> (element=w244:T2)
    n205 = Unbundle By Name(w244) -> ("Xmax"=w240:dbl, "Xmin"=w239:dbl, "Ymax"=w238:dbl, "Ymin"=w237:dbl, "Xc"=w236:dbl, "Yc"=w235:dbl, "Px"=w234:dbl, "Py"=w233:dbl, "q"=w232:dbl, "Level"=w214:i32)
    n206 = Increment(x=w212) -> (x+1=w219:i32)
    n207 = Increment(x=w210) -> (x+1=w206:i32)
    n208 = Increment(x=w147) -> (x+1=w151:i32)
    n209 = Increment(x=w142) -> (x+1=w138:i32)
    n210 = formula code="Xmax2 = Xmax ;\nXmin2 = Xc ;\nYmax2 = Ymax ;\nYmin2 = Yc ;\nXc2 = 0.5 * (Xmax + Xc) ;\nYc2 = 0.5 * (Ymax + Yc) ;\nPx2 = Px + L * sin(q + dqx2) ;\nPy2 = Py + L * cos(q + dqx2) ;\nq2 = q + dqx2 ;"("Xmax"=w240, "Xmin"=w239, "Ymax"=w238, "Ymin"=w237, "Xc"=w236, "Yc"=w235, "Px"=w234, "Py"=w233, "q"=w232, "dq"=w107, "dqx2"=w108, "L"=w106) -> ("Xmax2"=w222:dbl, "Xmin2"=w223:dbl, "Ymax2"=w224:dbl, "Ymin2"=w225:dbl, "Xc2"=w226:dbl, "Yc2"=w227:dbl, "Px2"=w228:dbl, "Py2"=w229:dbl, "q2"=w230:dbl)
    n211 = Greater?(x=w220, y=w219) -> (0:w218:bool)
    n212 = Greater?(x=w205, y=w206) -> (0:w207:bool)
    n213 = Greater?(x=w152, y=w151) -> (0:w150:bool)
    n214 = Greater?(x=w137, y=w138) -> (0:w139:bool)
    n215 = case shown="True" w218 {
      tunnel: w217 -> [_ w293]
      tunnel: w216 -> [w288 w292]
      tunnel: w215 -> [w287 w291]
      tunnel: [w288 w290] -> w178
      tunnel: [w287 w289] -> w177
      frame False {
      }
      frame True {
        n216 = Enqueue Element At Opposite End(queue=w292, element=w293, error in (no error)=w291) -> (queue out=w290:refnum<queue>, error out=w289:errorcluster)  [unwired: 2 out]
      }
    }
    n217 = Increment(x=w214) -> (x+1=w231:i32)
    n218 = Bundle By Name(cluster=w105, "Xmax"=w222, "Xmin"=w223, "Ymax"=w224, "Ymin"=w225, "Xc"=w226, "Yc"=w227, "Px"=w228, "Py"=w229, "q"=w230, "Level"=w231, "ObjIndexList"=w211, "ParentIndex"=w103, "NodeQ1Index"=w221, "NodeQ2Index"=w221, "NodeQ3Index"=w221, "NodeQ4Index"=w221) -> (w243:T4)
    n219 = call "Create_TreeNode_PN.vi"("Input cluster"=w243) -> ("TreeNode out"=w242:T2)
    n220 = Build Array (concatenate)(w241, w242) -> (w179:T2[])
    n221 = Array Size(array=w179) -> (size(s)=w208:i32)
    n222 = in-place {
      in-place-border: w208 -> [w285]
      n223 = in-place-array #2(w179, w103) -> (w286:T2)
      n224 = Bundle By Name(cluster=w286, "NodeQ2Index"=w285) -> (w284:T2)
      n225 = in-place-array #2(w284) -> (w184:T2[])  [unwired: 1 out]
    }
    n226 = Index Array(array=w184, index=w103) -> (element=w181:T2)
    n227 = Unbundle By Name(w181) -> ("Xmax"=w185:dbl, "Xmin"=w186:dbl, "Ymax"=w187:dbl, "Ymin"=w188:dbl, "Xc"=w189:dbl, "Yc"=w190:dbl, "Px"=w191:dbl, "Py"=w192:dbl, "q"=w193:dbl, "Level"=w209:i32)
    n228 = formula code="Xmax2 = Xc ;\nXmin2 = Xmin ;\nYmax2 = Ymax ;\nYmin2 = Yc ;\nXc2 = 0.5 * (Xc + Xmin) ;\nYc2 = 0.5 * (Ymax + Yc) ;\nPx2 = Px + L * sin(q + dq) ;\nPy2 = Py + L * cos(q + dq) ;\nq2 = q + dq ;"("Xmax"=w185, "Xmin"=w186, "Ymax"=w187, "Ymin"=w188, "Xc"=w189, "Yc"=w190, "Px"=w191, "Py"=w192, "q"=w193, "dq"=w107, "dqx2"=w108, "L"=w106) -> ("Xmax2"=w203:dbl, "Xmin2"=w202:dbl, "Ymax2"=w201:dbl, "Ymin2"=w200:dbl, "Xc2"=w199:dbl, "Yc2"=w198:dbl, "Px2"=w197:dbl, "Py2"=w196:dbl, "q2"=w195:dbl)
    n229 = case shown="True" w207 {
      tunnel: w208 -> [_ w283]
      tunnel: w178 -> [w278 w282]
      tunnel: w177 -> [w277 w281]
      tunnel: [w278 w280] -> w146
      tunnel: [w277 w279] -> w145
      frame False {
      }
      frame True {
        n230 = Enqueue Element At Opposite End(queue=w282, element=w283, error in (no error)=w281) -> (queue out=w280:refnum<queue>, error out=w279:errorcluster)  [unwired: 2 out]
      }
    }
    n231 = Increment(x=w209) -> (x+1=w194:i32)
    n232 = Bundle By Name(cluster=w105, "Xmax"=w203, "Xmin"=w202, "Ymax"=w201, "Ymin"=w200, "Xc"=w199, "Yc"=w198, "Px"=w197, "Py"=w196, "q"=w195, "Level"=w194, "ObjIndexList"=w180, "ParentIndex"=w103, "NodeQ1Index"=w204, "NodeQ2Index"=w204, "NodeQ3Index"=w204, "NodeQ4Index"=w204) -> (w182:T4)
    n233 = call "Create_TreeNode_PN.vi"("Input cluster"=w182) -> ("TreeNode out"=w183:T2)
    n234 = Build Array (concatenate)(w184, w183) -> (w144:T2[])
    n235 = Array Size(array=w144) -> (size(s)=w149:i32)
    n236 = in-place {
      in-place-border: w149 -> [w275]
      n237 = in-place-array #3(w144, w103) -> (w276:T2)
      n238 = Bundle By Name(cluster=w276, "NodeQ3Index"=w275) -> (w274:T2)
      n239 = in-place-array #3(w274) -> (w173:T2[])  [unwired: 1 out]
    }
    n240 = Index Array(array=w173, index=w103) -> (element=w176:T2)
    n241 = Unbundle By Name(w176) -> ("Xmax"=w172:dbl, "Xmin"=w171:dbl, "Ymax"=w170:dbl, "Ymin"=w169:dbl, "Xc"=w168:dbl, "Yc"=w167:dbl, "Px"=w166:dbl, "Py"=w165:dbl, "q"=w164:dbl, "Level"=w148:i32)
    n242 = formula code="Xmax2 = Xc ;\nXmin2 = Xmin ;\nYmax2 = Yc ;\nYmin2 = Ymin ;\nXc2 = 0.5 * (Xc + Xmin) ;\nYc2 = 0.5 * (Yc + Ymin) ;\nPx2 = Px + L * sin(q - dq) ;\nPy2 = Py + L * cos(q - dq) ;\nq2 = q - dq ;"("Xmax"=w172, "Xmin"=w171, "Ymax"=w170, "Ymin"=w169, "Xc"=w168, "Yc"=w167, "Px"=w166, "Py"=w165, "q"=w164, "dq"=w107, "dqx2"=w108, "L"=w106) -> ("Xmax2"=w154:dbl, "Xmin2"=w155:dbl, "Ymax2"=w156:dbl, "Ymin2"=w157:dbl, "Xc2"=w158:dbl, "Yc2"=w159:dbl, "Px2"=w160:dbl, "Py2"=w161:dbl, "q2"=w162:dbl)
    n243 = case shown="True" w150 {
      tunnel: w149 -> [_ w273]
      tunnel: w146 -> [w268 w272]
      tunnel: w145 -> [w267 w271]
      tunnel: [w268 w270] -> w110
      tunnel: [w267 w269] -> w111
      frame False {
      }
      frame True {
        n244 = Enqueue Element At Opposite End(queue=w272, element=w273, error in (no error)=w271) -> (queue out=w270:refnum<queue>, error out=w269:errorcluster)  [unwired: 2 out]
      }
    }
    n245 = Increment(x=w148) -> (x+1=w163:i32)
    n246 = Bundle By Name(cluster=w105, "Xmax"=w154, "Xmin"=w155, "Ymax"=w156, "Ymin"=w157, "Xc"=w158, "Yc"=w159, "Px"=w160, "Py"=w161, "q"=w162, "Level"=w163, "ObjIndexList"=w143, "ParentIndex"=w103, "NodeQ1Index"=w153, "NodeQ2Index"=w153, "NodeQ3Index"=w153, "NodeQ4Index"=w153) -> (w175:T4)
    n247 = call "Create_TreeNode_PN.vi"("Input cluster"=w175) -> ("TreeNode out"=w174:T2)
    n248 = Build Array (concatenate)(w173, w174) -> (w109:T2[])
    n249 = Array Size(array=w109) -> (size(s)=w140:i32)
    n250 = in-place {
      in-place-border: w140 -> [w265]
      n251 = in-place-array #4(w109, w103) -> (w266:T2)
      n252 = Bundle By Name(cluster=w266, "NodeQ4Index"=w265) -> (w264:T2)
      n253 = in-place-array #4(w264) -> (w116:T2[])  [unwired: 1 out]
    }
    n254 = Index Array(array=w116, index=w103) -> (element=w113:T2)
    n255 = Unbundle By Name(w113) -> ("Xmax"=w117:dbl, "Xmin"=w118:dbl, "Ymax"=w119:dbl, "Ymin"=w120:dbl, "Xc"=w121:dbl, "Yc"=w122:dbl, "Px"=w123:dbl, "Py"=w124:dbl, "q"=w125:dbl, "Level"=w141:i32)
    n256 = formula code="Xmax2 = Xmax ;\nXmin2 = Xc ;\nYmax2 = Yc ;\nYmin2 = Ymin ;\nXc2 = 0.5 * (Xmax + Xc) ;\nYc2 = 0.5 * (Yc + Ymin) ;\nPx2 = Px + L * sin(q - dqx2) ;\nPy2 = Py + L * cos(q - dqx2) ;\nq2 = q - dqx2 ;"("Xmax"=w117, "Xmin"=w118, "Ymax"=w119, "Ymin"=w120, "Xc"=w121, "Yc"=w122, "Px"=w123, "Py"=w124, "q"=w125, "dq"=w107, "dqx2"=w108, "L"=w106) -> ("Xmax2"=w135:dbl, "Xmin2"=w134:dbl, "Ymax2"=w133:dbl, "Ymin2"=w132:dbl, "Xc2"=w131:dbl, "Yc2"=w130:dbl, "Px2"=w129:dbl, "Py2"=w128:dbl, "q2"=w127:dbl)
    n257 = case shown="True" w139 {
      tunnel: w140 -> [_ w263]
      tunnel: w110 -> [w258 w262]
      tunnel: w111 -> [w257 w261]
      tunnel: [w258 w260] -> w102
      tunnel: [w257 w259] -> w101
      frame False {
      }
      frame True {
        n258 = Enqueue Element At Opposite End(queue=w262, element=w263, error in (no error)=w261) -> (queue out=w260:refnum<queue>, error out=w259:errorcluster)  [unwired: 2 out]
      }
    }
    n259 = Increment(x=w141) -> (x+1=w126:i32)
    n260 = Bundle By Name(cluster=w105, "Xmax"=w135, "Xmin"=w134, "Ymax"=w133, "Ymin"=w132, "Xc"=w131, "Yc"=w130, "Px"=w129, "Py"=w128, "q"=w127, "Level"=w126, "ObjIndexList"=w104, "ParentIndex"=w103, "NodeQ1Index"=w136, "NodeQ2Index"=w136, "NodeQ3Index"=w136, "NodeQ4Index"=w136) -> (w114:T4)
    n261 = call "Create_TreeNode_PN.vi"("Input cluster"=w114) -> ("TreeNode out"=w115:T2)
    n262 = Build Array (concatenate)(w116, w115) -> (w94:T2[])
    n263 = Get Queue Status(queue=w102, error in (no error)=w101) -> (queue out=w254:refnum<queue>, error out=w253:errorcluster, # elements in queue=w100:i32)  [unwired: 6 out]
    n264 = Equal To 0?(x=w100) -> (x = 0?=w98:bool)
    n265 = Or(x=w98, y="stop") -> (x .or. y?=w97:bool)
    n266 = Build Array (concatenate)(w93, w100) -> (w99:i32[])
    "Node stack size history" <- w93
  }
  "Node stack size history" <- w10
  "TreeNodes out" <- w11
  n267 = disable-structure shown="Disabled" {
    disable-tunnel: w10 -> [w831 _]
    frame Disabled {
      n268 = call-poly <vilib>:"Write To Spreadsheet File.vi"("transpose? (no:F)"=TRUE, "1D data"=w831) -> ()  [unwired: 4 in, 3 out]
    }
    frame Enabled {
    }
  }
  n269 = for {
    tunnel: w11 -> [w834] mode=indexing
    tunnel: [w833] -> w13 mode=indexing
    tunnel: [w832] -> w12 mode=indexing
    n270 = Unbundle By Name(w834) -> ("Px"=w833:dbl, "Py"=w832:dbl)
  }
  n271 = Unbundle By Name(w23) -> ("status"=w22:bool)
  n272 = Release Queue(queue=w29, error in (no error)=w23) -> ()  [unwired: 4 out]
  n273 = Array Size(array=w10) -> (size(s)=w18:i32)
  n274 = Decrement(x=w18) -> (x-1=w24:i32)
  n275 = Index Array(array=w10, index=w24) -> (element=w16:i32)
  n276 = Bundle(w13, w12) -> (→"Node tree representation":cluster{dbl[], dbl[]})  [unwired: 1 out]
  n277 = Equal To 0?(x=w16) -> (x = 0?=w20:bool)
  n278 = Not(x=w22) -> (.not. x?=w21:bool)
  n279 = And(x=w21, y=w20) -> (x .and. y?=→"All nodes processed and processed without error":bool)
  n280 = local write "Node stack size history"(w10) -> ()
